vi "ReadSMUBuffer.vi"(7 "SMU":T2, 8 "Error In":errorcluster, 10 "Measure Configuration":T1={"Enabled?"=FALSE, "Count"=1, "Interval (sec)"=0.025, "Voltage Auto Range Enabled?"=TRUE, "Voltage High Limit (V or A)"=0.0, "Voltage Low Limit (V or A)"=0.0, "Current Auto Range Enabled?"=TRUE, "Current High Limit (V or A)"=0.0, "Current Low Limit (V or A)"=0.0} {"Count" min=1 step=1}, 11 "Kiethley 2602 In":refnum<visa-resource-name>) -> (0 "Error Out":errorcluster, 2 "Data":dbl[](array[numeric]), 3 "Keithley 2602 Out":refnum<visa-resource-name>)   [LabVIEW 2012]
uses:
  driver/Public/Controls/SMU.ctl
  MeasureConfiguration.ctl
  driver/Public/Controls/BufferValue.ctl
  <vilib>/Analysis/baseanly.llb/Mean (DBL).vi
  driver/Keithley-2602.lvlib
  libs/LV-Utilities/LV-Utilities.lvlib
  <vilib>/Analysis/NI_AALBase.lvlib
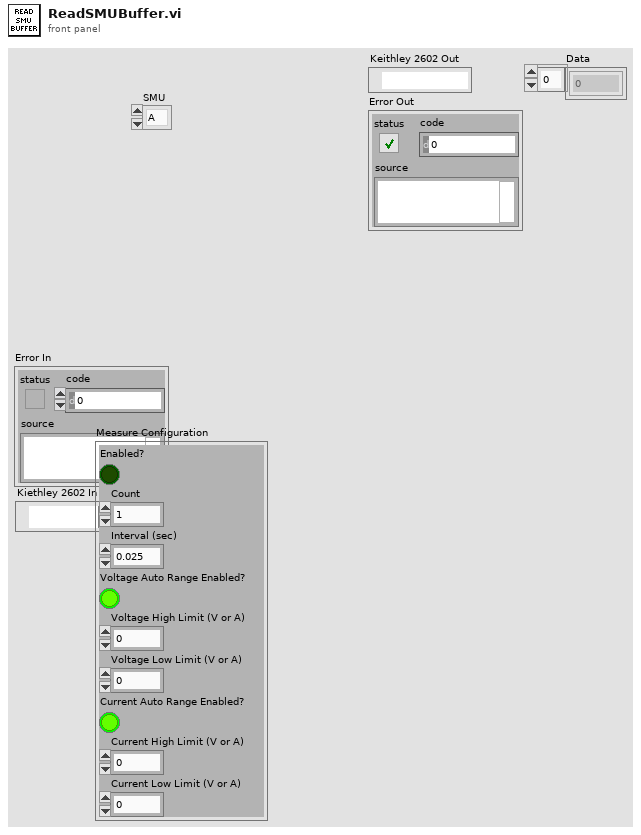
[diagram p1: front panel]
types:
  T1 = typedef "MeasureConfiguration.ctl" = cluster{"Enabled?":bool, "Count":u8, "Interval (sec)":dbl, "Voltage Auto Range Enabled?":bool, "Voltage High Limit (V or A)":dbl, "Voltage Low Limit (V or A)":dbl, "Current Auto Range Enabled?":bool, "Current High Limit (V or A)":dbl, "Current Low Limit (V or A)":dbl}
  T2 = typedef "Keithley-2602.lvlib/SMU.ctl" = enum16{"A", "B"}
  T3 = typedef "Keithley-2602.lvlib/BufferValue.ctl" = enum16{"Readings", "Source", "Timestamp"}
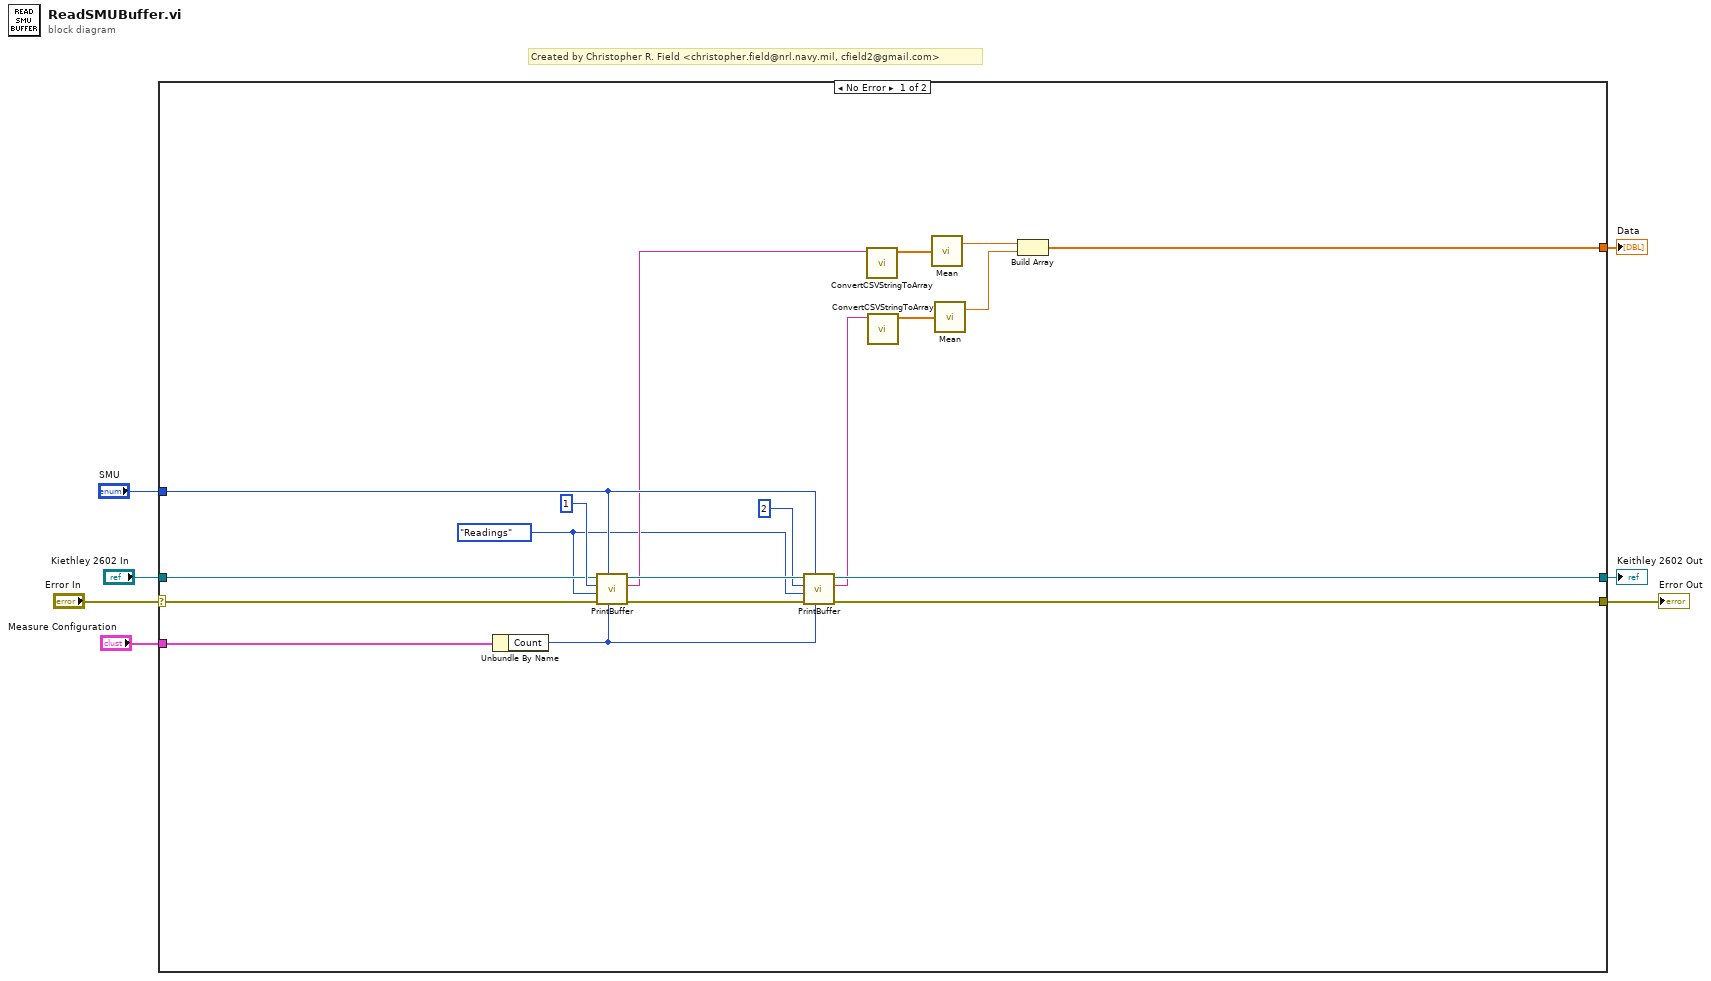
[diagram p0: block diagram]
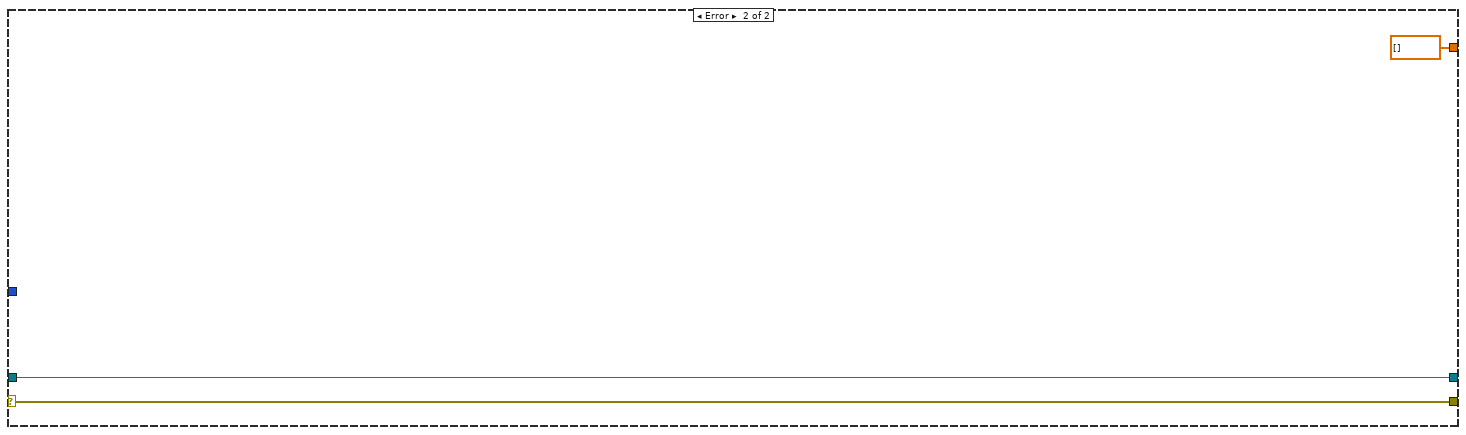
[diagram p2: hidden frame]
diagram:
  # "Created by Christopher R. Field <christopher.field@nrl.navy.mil, cfield2@gmail.com>"
  n1 = case shown="No Error" "Error In" {
    selector: "Error In" -> [w21 w29]
    tunnel: "Kiethley 2602 In" -> [w22 w28]
    tunnel: "Measure Configuration" -> [w20 _]
    tunnel: [w18 w28] -> w5
    tunnel: [w17 w29] -> w4
    tunnel: "SMU" -> [w16 _]
    tunnel: [w8 dbl[] []] -> w1
    frame No Error {
      w13 = BufferValue."Readings" ("Buffer Value")
      n2 = Unbundle By Name(w20) -> ("Count"=w19:u8)
      n3 = call "PrintBuffer.vi"("Number of Data Points"=w19, "SMU"=w16, "Error In"=w21, "Buffer Value"=w13, "Buffer"=u8 1, "Kiethley 2602 In"=w22) -> ("Error Out"=w25:errorcluster, "Buffer"=w15:string, "Keithley 2602 Out"=w26:refnum<visa-resource-name>)  [unwired: 3 in]
      n4 = call "PrintBuffer.vi"("Number of Data Points"=w19, "SMU"=w16, "Error In"=w25, "Buffer Value"=w13, "Buffer"=u8 2, "Kiethley 2602 In"=w26) -> ("Error Out"=w17:errorcluster, "Buffer"=w14:string, "Keithley 2602 Out"=w18:refnum<visa-resource-name>)  [unwired: 3 in]
      n5 = call "ConvertCSVStringToArray.vi"("CSV String"=w15) -> ("Array"=w12:dbl[])  [unwired: 10 in]
      n6 = call "ConvertCSVStringToArray.vi"("CSV String"=w14) -> ("Array"=w11:dbl[])  [unwired: 10 in]
      n7 = call-poly <vilib>:"Mean.vi"("X"=w12) -> ("mean"=w10:dbl)  [unwired: 1 out]
      n8 = call-poly <vilib>:"Mean.vi"("X"=w11) -> ("mean"=w9:dbl)  [unwired: 1 out]
      n9 = Build Array(w10, w9) -> (w8:dbl[])
    }
    frame Error {
    }
  }
  "Keithley 2602 Out" <- w5
  "Error Out" <- w4
  "Data" <- w1
